vi "Load Controls.vi"(8 "Parent Label":string, 9 "Parent Class":string, 10 "Controls[]":refnum<vi>[](array[refnum]), 11 "Ref Config File In":T1) -> (3 "Ref Config File Out":T1)   [LabVIEW 2009]
uses:
  <vilib>/Utility/config.llb/Config Data RefNum.ctl
  <vilib>/Utility/config.llb/Read Key (Double).vi
  <vilib>/Utility/config.llb/Read Key (Boolean).vi
  <vilib>/Utility/config.llb/Read Key (String).vi
  <vilib>/Utility/config.llb/Read Key (Path).vi
  <vilib>/Utility/config.llb/Read Key (I32).vi
  <vilib>/Utility/config.llb/NI_LVConfig.lvlib
panel:
  # "Guillaume Plateau - Dec. 9, 2009\nyguig2@yahoo.fr - Version 3.0"
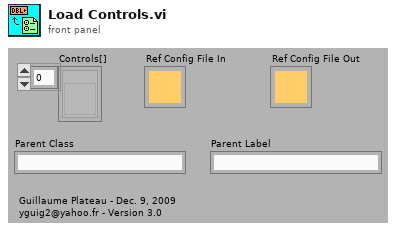
[diagram p1: front panel]
types:
  T1 = typedef "NI_LVConfig.lvlib/Config Data RefNum.ctl" = refnum<k1>
  T2 = typedef "LVCursorListTypeDef.ctl" = cluster{"Name":string, "Color":u32, "Style":u8, "Point Style":u8, "Name Visible":bool, "Allow Drag":bool, "Cursor Mode":u32, "Plot":i32, "Index":i32, "Position":cluster{"X":dbl, "Y":dbl}, "X Scale":u32, "Y Scale":u32, "Watch Plots":i32[], "Watch All Plots":bool, "Plot Area":i32, "Label Offset":cluster{"X":dbl, "Y":dbl}}[]
  T3 = cluster{"Name":string, "Color":u32, "Style":u8, "Point Style":u8, "Name Visible":bool, "Allow Drag":bool, "Cursor Mode":u32, "Plot":i32, "Index":i32, "Position":cluster{"X":dbl, "Y":dbl}, "X Scale":u32, "Y Scale":u32, "Watch Plots":i32[], "Watch All Plots":bool, "Plot Area":i32, "Label Offset":cluster{"X":dbl, "Y":dbl}}
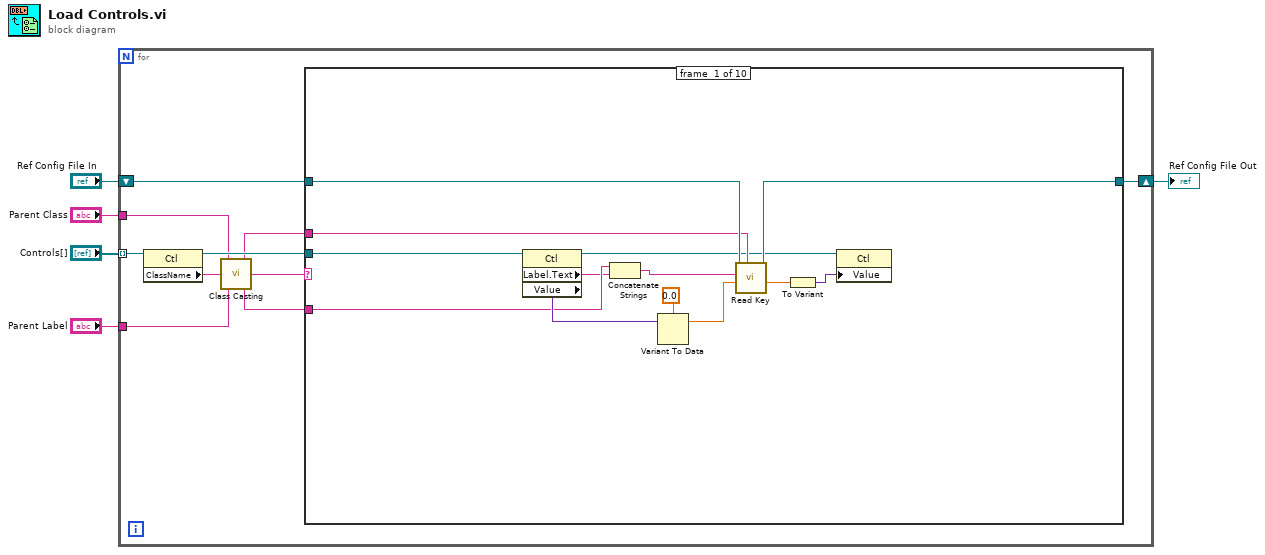
[diagram p0: block diagram]
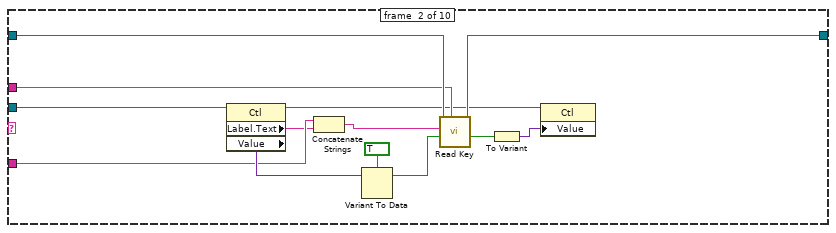
[diagram p2: hidden frame]
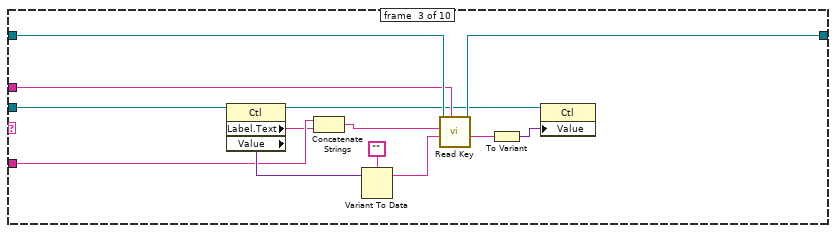
[diagram p3: hidden frame]
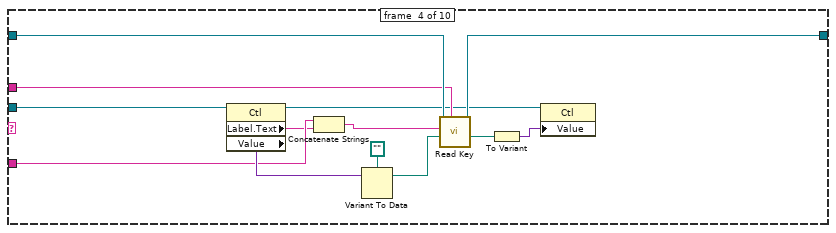
[diagram p4: hidden frame]
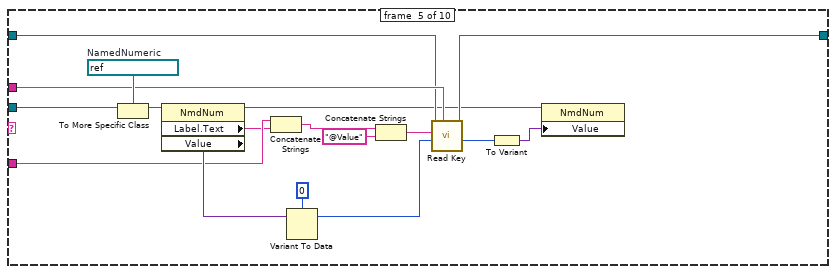
[diagram p5: hidden frame]
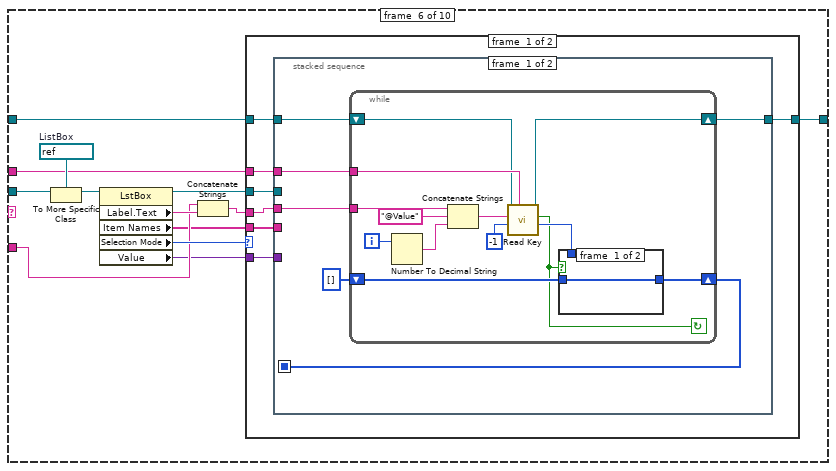
[diagram p6: hidden frame]
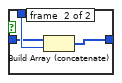
[diagram p7: hidden frame]
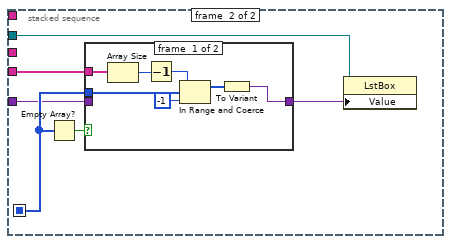
[diagram p8: hidden frame]
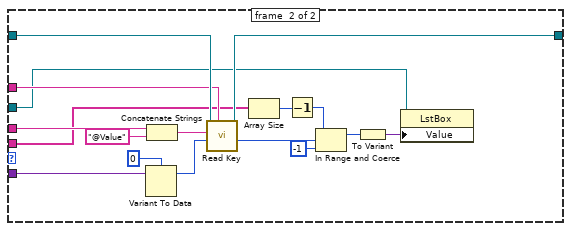
[diagram p10: hidden frame]
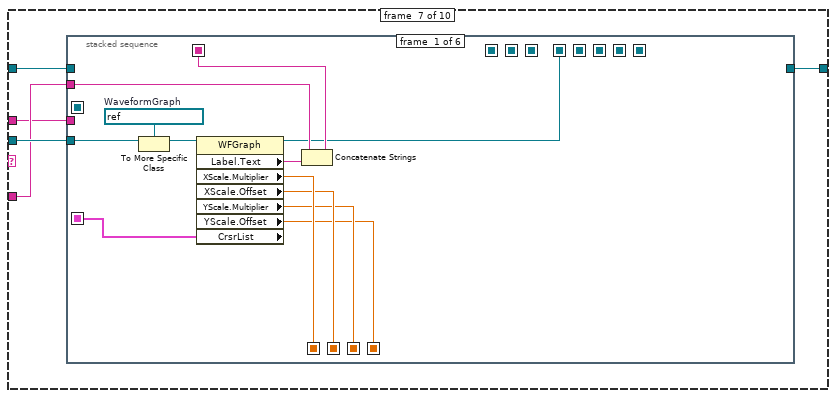
[diagram p11: hidden frame]
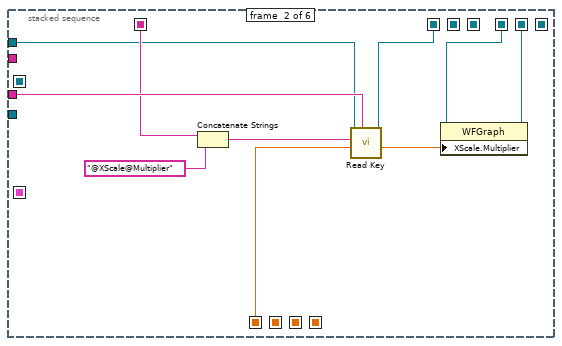
[diagram p12: hidden frame]
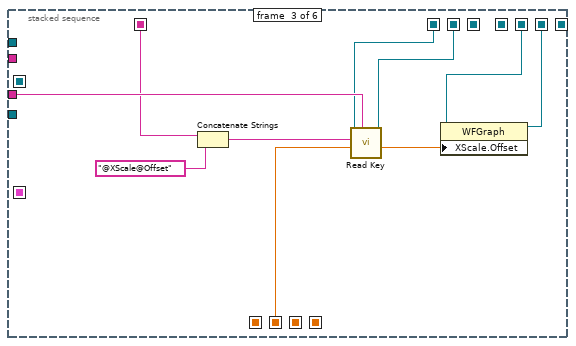
[diagram p13: hidden frame]
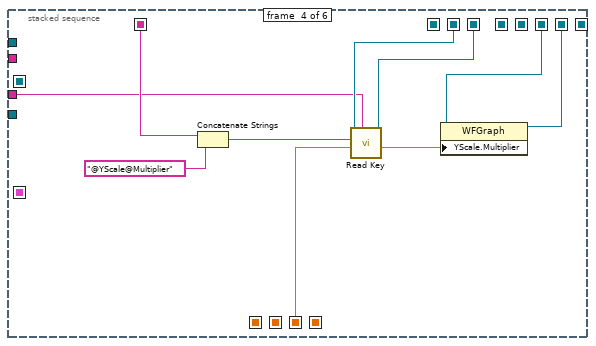
[diagram p14: hidden frame]
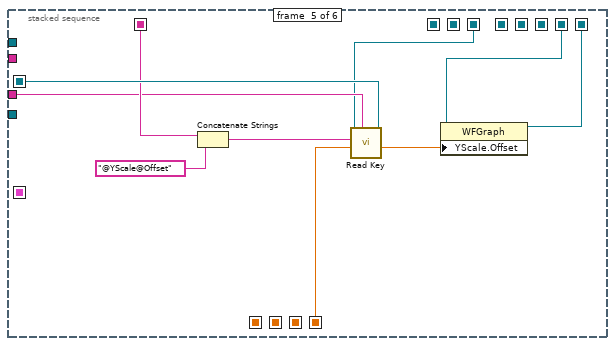
[diagram p15: hidden frame]
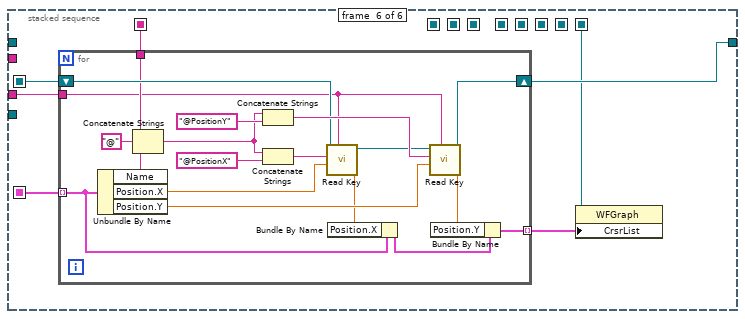
[diagram p16: hidden frame]
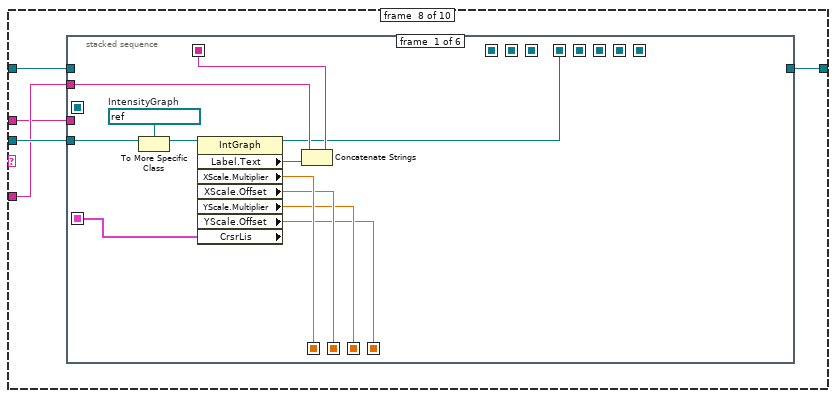
[diagram p17: hidden frame]
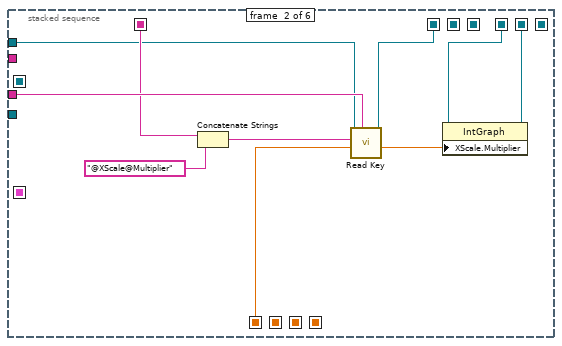
[diagram p18: hidden frame]
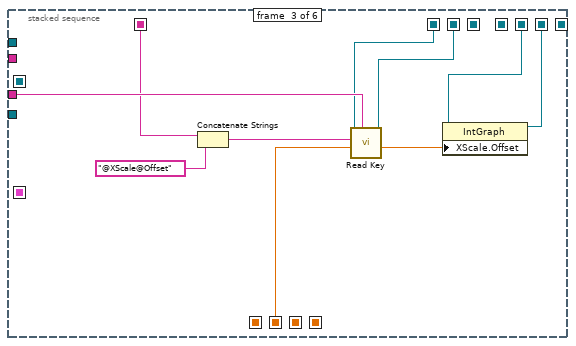
[diagram p19: hidden frame]
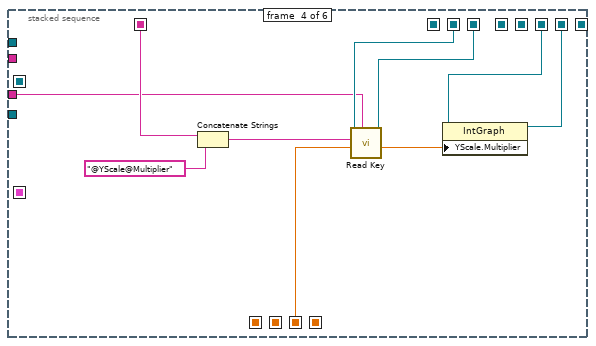
[diagram p20: hidden frame]
diagram:
  n1 = for {
    tunnel: "Controls[]" -> [w12] mode=indexing
    shift-right: [w13] -> w5
    shift-left: "Ref Config File In" -> [w14]
    tunnel: "Parent Class" -> [w7]
    tunnel: "Parent Label" -> [w11]
    n2 = property class="Ctl"(reference=w12) -> (reference out=w9:refnum<vi>, "ClassName"=w8:string)  [unwired: 1 in, 1 out]
    n3 = call "Class Casting.vi"("Parent Label"=w11, "Control Class"=w8, "Parent Class"=w7) -> ("Add-on Label"=w10:string, "Class"=w6:string)  [unwired: 1 out]
    n4 = case shown="\"WaveformGraph\"" w8 {
      tunnel: w9 -> [w15 w39 w52 w65 w82 w96 w162 w245 w328 _]
      tunnel: w14 -> [w25 w37 w50 w63 w71 w92 w161 w244 w327 w407]
      tunnel: [w24 w36 w49 w62 w83 w91 w160 w243 w326 w407] -> w13
      tunnel: w10 -> [w23 w34 w47 w60 w75 w88 w159 w242 w325 _]
      tunnel: w6 -> [w20 w32 w45 w58 w72 w87 w158 w241 w324 _]
      frame #0 {
        n5 = property class="Ctl"(reference=w15) -> (reference out=w18:refnum<vi>, "Label.Text"=w21:string, "Value"=w26:variant)  [unwired: 1 in, 1 out]
        n6 = Concatenate Strings(w23, w21) -> (w22:string)
        n7 = Variant To Data(Variant=w26, type=0.0) -> (data=w19:dbl)  [unwired: 1 in, 1 out]
        n8 = call-poly <vilib>:"Read Key.vi"("section"=w20, "default value"=w19, "key"=w22, "refnum"=w25) -> ("value"=w17:dbl, "refnum out"=w24:T1)  [unwired: 3 in, 3 out]
        n9 = To Variant(anything=w17) -> (Variant=w16:variant)
        n10 = property class="Ctl"(reference=w18, "Value"=w16) -> ()  [unwired: 1 in, 2 out]
      }
      frame #1 {
        n11 = property class="Ctl"(reference=w39) -> (reference out=w28:refnum<vi>, "Label.Text"=w33:string, "Value"=w38:variant)  [unwired: 1 in, 1 out]
        n12 = Concatenate Strings(w34, w33) -> (w35:string)
        n13 = Variant To Data(Variant=w38, type=TRUE) -> (data=w31:bool)  [unwired: 1 in, 1 out]
        n14 = call-poly <vilib>:"Read Key.vi"("section"=w32, "default value"=w31, "key"=w35, "refnum"=w37) -> ("value"=w29:bool, "refnum out"=w36:T1)  [unwired: 1 in, 5 out]
        n15 = To Variant(anything=w29) -> (Variant=w30:variant)
        n16 = property class="Ctl"(reference=w28, "Value"=w30) -> ()  [unwired: 1 in, 2 out]
      }
      frame #2 {
        n17 = property class="Ctl"(reference=w52) -> (reference out=w41:refnum<vi>, "Label.Text"=w46:string, "Value"=w51:variant)  [unwired: 1 in, 1 out]
        n18 = Concatenate Strings(w47, w46) -> (w48:string)
        n19 = Variant To Data(Variant=w51, type="") -> (data=w44:string)  [unwired: 1 in, 1 out]
        n20 = call-poly <vilib>:"Read Key.vi"("section"=w45, "default value"=w44, "key"=w48, "refnum"=w50) -> ("value"=w42:string, "refnum out"=w49:T1)  [unwired: 2 in, 4 out]
        n21 = To Variant(anything=w42) -> (Variant=w43:variant)
        n22 = property class="Ctl"(reference=w41, "Value"=w43) -> ()  [unwired: 1 in, 2 out]
      }
      frame #3 {
        n23 = property class="Ctl"(reference=w65) -> (reference out=w54:refnum<vi>, "Label.Text"=w59:string, "Value"=w64:variant)  [unwired: 1 in, 1 out]
        n24 = Concatenate Strings(w60, w59) -> (w61:string)
        n25 = Variant To Data(Variant=w64, type=path "") -> (data=w57:path)  [unwired: 1 in, 1 out]
        n26 = call-poly <vilib>:"Read Key.vi"("section"=w58, "default value"=w57, "key"=w61, "refnum"=w63) -> ("value"=w55:path, "refnum out"=w62:T1)  [unwired: 1 in, 5 out]
        n27 = To Variant(anything=w55) -> (Variant=w56:variant)
        n28 = property class="Ctl"(reference=w54, "Value"=w56) -> ()  [unwired: 1 in, 2 out]
      }
      frame #4 {
        w81 = refnum<vi> refnum  # NamedNumeric
        n29 = To More Specific Class(target class=w81, reference=w82) -> (specific class reference=w80:refnum<vi>)  [unwired: 1 in, 1 out]
        n30 = property class="NmdNum"(reference=w80) -> (reference out=w67:refnum<vi>, "Label.Text"=w74:string, "Value"=w78:variant)  [unwired: 1 in, 1 out]
        n31 = Concatenate Strings(w75, w74) -> (w73:string)
        n32 = Variant To Data(Variant=w78, type=0) -> (data=w69:i32)  [unwired: 1 in, 1 out]
        n33 = Concatenate Strings(w73, "@Value" ("string")) -> (w76:string)
        n34 = call-poly <vilib>:"Read Key.vi"("section"=w72, "default value"=w69, "key"=w76, "refnum"=w71) -> ("value"=w68:i32, "refnum out"=w83:T1)  [unwired: 1 in, 5 out]
        n35 = To Variant(anything=w68) -> (Variant=w70:variant)
        n36 = property class="NmdNum"(reference=w67, "Value"=w70) -> ()  [unwired: 1 in, 2 out]
      }
      frame #5 {
        w95 = refnum<vi> refnum  # ListBox
        n37 = To More Specific Class(target class=w95, reference=w96) -> (specific class reference=w94:refnum<vi>)  [unwired: 1 in, 1 out]
        n38 = property class="LstBox"(reference=w94) -> (reference out=w85:refnum<vi>, "Label.Text"=w90:string, "Item Names"=w86:string[], "Selection Mode"=w93:i32, "Value"=w84:variant)  [unwired: 1 in, 1 out]
        n39 = Concatenate Strings(w88, w90) -> (w89:string)
        n40 = case shown="0, 1, Default" w93 {
          tunnel: w92 -> [w103 w157]
          tunnel: w87 -> [w102 w156]
          tunnel: w89 -> [w101 w155]
          tunnel: [w100 w154] -> w91
          tunnel: w86 -> [w99 w143]
          tunnel: w85 -> [w97 w141]
          tunnel: w84 -> [w98 w150]
          frame #0 {
            n41 = stacked-sequence {
              seq-local: [w104 _] -> [_ w131]
              tunnel: w103 -> [w109 _]
              tunnel: w102 -> [w108 _]
              tunnel: w101 -> [w107 _]
              tunnel: [w106 _] -> w100
              tunnel: w99 -> [_ w130]
              tunnel: w98 -> [_ w129]
              tunnel: w97 -> [_ w127]
              frame #0 {
                n42 = while {
                  shift-right: [w118] -> w106
                  shift-left: w109 -> [w115]
                  tunnel: w108 -> [w116]
                  tunnel: w107 -> [w117]
                  shift-right: [w111] -> w104
                  shift-left: i32[] [] -> [w112]
                  i -> [w120]
                  stop <- w110 continue-if-true
                  n43 = Number To Decimal String(number=w120) -> (decimal integer string=w119:string)  [unwired: 1 out]
                  n44 = Concatenate Strings(w117, "@Value" ("string"), w119) -> (w121:string)
                  n45 = call-poly <vilib>:"Read Key.vi"("section"=w116, "default value"=-1, "key"=w121, "refnum"=w115) -> ("value"=w113:i32, "found?"=w110:bool, "refnum out"=w118:T1)  [unwired: 1 in, 4 out]
                  n46 = case shown="True" w110 {
                    tunnel: w113 -> [_ w126]
                    tunnel: w112 -> [w123 w125]
                    tunnel: [w123 w124] -> w111
                    frame #0 {
                    }
                    frame #1 {
                      n47 = Build Array (concatenate)(w125, w126) -> (w124:i32[])
                    }
                  }
                }
              }
              frame #1 {
                n48 = Empty Array?(array=w131) -> (empty?=w132:bool)
                n49 = case shown="False" w132 {
                  tunnel: w131 -> [w135 _]
                  tunnel: w130 -> [w134 _]
                  tunnel: [w133 w140] -> w128
                  tunnel: w129 -> [_ w140]
                  frame #0 {
                    n50 = Array Size(array=w134) -> (size(s)=w138:i32)
                    n51 = Decrement(x=w138) -> (x-1=w137:i32)
                    n52 = In Range and Coerce(upper limit=w137, x=w135, lower limit=-1) -> (coerced(x)=w136:i32[])  [unwired: 1 out]
                    n53 = To Variant(anything=w136) -> (Variant=w133:variant)
                  }
                  frame #1 {
                  }
                }
                n54 = property class="LstBox"(reference=w127, "Value"=w128) -> ()  [unwired: 1 in, 2 out]
              }
            }
          }
          frame #1 {
            n55 = Variant To Data(Variant=w150, type=0) -> (data=w149:i32)  [unwired: 1 in, 1 out]
            n56 = Concatenate Strings(w155, "@Value" ("string")) -> (w152:string)
            n57 = call-poly <vilib>:"Read Key.vi"("section"=w156, "default value"=w149, "key"=w152, "refnum"=w157) -> ("value"=w144:i32, "refnum out"=w154:T1)  [unwired: 1 in, 5 out]
            n58 = Array Size(array=w143) -> (size(s)=w147:i32)
            n59 = Decrement(x=w147) -> (x-1=w146:i32)
            n60 = In Range and Coerce(upper limit=w146, x=w144, lower limit=-1) -> (coerced(x)=w145:i32)  [unwired: 1 out]
            n61 = To Variant(anything=w145) -> (Variant=w142:variant)
            n62 = property class="LstBox"(reference=w141, "Value"=w142) -> ()  [unwired: 1 in, 2 out]
          }
        }
      }
      frame #6 {
        n63 = stacked-sequence {
          seq-local: [w171 _ _ _ _ _] -> [_ _ _ _ _ w221]
          seq-local: [_ _ _ _ w212 _] -> [_ _ _ _ _ w220]
          seq-local: [w170 _ _ _ _ _] -> [_ w180 _ _ _ _]
          seq-local: [w169 _ _ _ _ _] -> [_ _ w189 _ _ _]
          seq-local: [w168 _ _ _ _ _] -> [_ _ _ w198 _ _]
          seq-local: [w167 _ _ _ _ _] -> [_ _ _ _ w209 _]
          seq-local: [_ w176 _ _ _ _] -> [_ _ w188 _ _ _]
          seq-local: [_ _ w192 _ _ _] -> [_ _ _ w202 _ _]
          seq-local: [_ _ _ w201 _ _] -> [_ _ _ _ w206 _]
          seq-local: [w164 _ _ _ _ _] -> [_ w181 w190 w200 w211 w218]
          seq-local: [w163 _ _ _ _ _] -> [_ w175 _ _ _ _]
          seq-local: [_ w177 _ _ _ _] -> [_ _ w187 _ _ _]
          seq-local: [_ _ w185 _ _ _] -> [_ _ _ w197 _ _]
          seq-local: [_ _ _ w195 _ _] -> [_ _ _ _ w205 _]
          seq-local: [_ _ _ _ w207 _] -> [_ _ _ _ _ w215]
          tunnel: w162 -> [w172 _ _ _ _ _]
          tunnel: w161 -> [_ w178 _ _ _ _]
          tunnel: [_ _ _ _ _ w219] -> w160
          tunnel: w158 -> [_ w182 w191 w199 w210 w217]
          tunnel: w159 -> [w165 _ _ _ _ _]
          frame #0 {
            w174 = refnum<vi> refnum  # WaveformGraph
            n64 = To More Specific Class(target class=w174, reference=w172) -> (specific class reference=w173:refnum<vi>)  [unwired: 1 in, 1 out]
            n65 = property class="WFGraph"(reference=w173) -> (reference out=w163:refnum<vi>, "Label.Text"=w166:string, "XScale.Multiplier"=w170:dbl, "XScale.Offset"=w169:dbl, "YScale.Multiplier"=w168:dbl, "YScale.Offset"=w167:dbl, "CrsrList"=w171:T2)  [unwired: 1 in, 1 out]
            n66 = Concatenate Strings(w165, w166) -> (w164:string)
          }
          frame #1 {
            n67 = Concatenate Strings(w181, "@XScale@Multiplier" ("string")) -> (w183:string)
            n68 = call-poly <vilib>:"Read Key.vi"("section"=w182, "default value"=w180, "key"=w183, "refnum"=w178) -> ("value"=w179:dbl, "refnum out"=w176:T1)  [unwired: 1 in, 5 out]
            n69 = property class="WFGraph"(reference=w175, "XScale.Multiplier"=w179) -> (reference out=w177:refnum<vi>)  [unwired: 1 in, 1 out]
          }
          frame #2 {
            n70 = Concatenate Strings(w190, "@XScale@Offset" ("string")) -> (w193:string)
            n71 = call-poly <vilib>:"Read Key.vi"("section"=w191, "default value"=w189, "key"=w193, "refnum"=w188) -> ("value"=w186:dbl, "refnum out"=w192:T1)  [unwired: 1 in, 5 out]
            n72 = property class="WFGraph"(reference=w187, "XScale.Offset"=w186) -> (reference out=w185:refnum<vi>)  [unwired: 1 in, 1 out]
          }
          frame #3 {
            n73 = Concatenate Strings(w200, "@YScale@Multiplier" ("string")) -> (w203:string)
            n74 = call-poly <vilib>:"Read Key.vi"("section"=w199, "default value"=w198, "key"=w203, "refnum"=w202) -> ("value"=w196:dbl, "refnum out"=w201:T1)  [unwired: 1 in, 5 out]
            n75 = property class="WFGraph"(reference=w197, "YScale.Multiplier"=w196) -> (reference out=w195:refnum<vi>)  [unwired: 1 in, 1 out]
          }
          frame #4 {
            n76 = Concatenate Strings(w211, "@YScale@Offset" ("string")) -> (w213:string)
            n77 = call-poly <vilib>:"Read Key.vi"("section"=w210, "default value"=w209, "key"=w213, "refnum"=w206) -> ("value"=w208:dbl, "refnum out"=w212:T1)  [unwired: 1 in, 5 out]
            n78 = property class="WFGraph"(reference=w205, "YScale.Offset"=w208) -> (reference out=w207:refnum<vi>)  [unwired: 1 in, 1 out]
          }
          frame #5 {
            n79 = for {
              shift-right: [w231] -> w219
              shift-left: w220 -> [w232]
              tunnel: w221 -> [w224] mode=indexing
              tunnel: w218 -> [w230]
              tunnel: w217 -> [w229]
              tunnel: [w222] -> w216 mode=indexing
              n80 = Unbundle By Name(w224) -> ("Name"=w239:string, "Position.X"=w228:dbl, "Position.Y"=w227:dbl)
              n81 = Concatenate Strings(w230, "@" ("string"), w239) -> (w233:string)
              n82 = Concatenate Strings(w233, "@PositionY" ("string")) -> (w235:string)
              n83 = Concatenate Strings(w233, "@PositionX" ("string")) -> (w236:string)
              n84 = call-poly <vilib>:"Read Key.vi"("section"=w229, "default value"=w228, "key"=w236, "refnum"=w232) -> ("value"=w226:dbl, "refnum out"=w234:T1)  [unwired: 1 in, 5 out]
              n85 = Bundle By Name(cluster=w224, "Position.X"=w226) -> (w223:T3)
              n86 = call-poly <vilib>:"Read Key.vi"("section"=w229, "default value"=w227, "key"=w235, "refnum"=w234) -> ("value"=w225:dbl, "refnum out"=w231:T1)  [unwired: 1 in, 5 out]
              n87 = Bundle By Name(cluster=w223, "Position.Y"=w225) -> (w222:T3)
            }
            n88 = property class="WFGraph"(reference=w215, "CrsrList"=w216) -> ()  [unwired: 1 in, 2 out]
          }
        }
      }
      frame #7 {
        n89 = stacked-sequence {
          seq-local: [w254 _ _ _ _ _] -> [_ _ _ _ _ w304]
          seq-local: [_ _ _ _ w295 _] -> [_ _ _ _ _ w303]
          seq-local: [w253 _ _ _ _ _] -> [_ w263 _ _ _ _]
          seq-local: [w252 _ _ _ _ _] -> [_ _ w272 _ _ _]
          seq-local: [w251 _ _ _ _ _] -> [_ _ _ w281 _ _]
          seq-local: [w250 _ _ _ _ _] -> [_ _ _ _ w292 _]
          seq-local: [_ w259 _ _ _ _] -> [_ _ w271 _ _ _]
          seq-local: [_ _ w275 _ _ _] -> [_ _ _ w285 _ _]
          seq-local: [_ _ _ w284 _ _] -> [_ _ _ _ w289 _]
          seq-local: [w247 _ _ _ _ _] -> [_ w264 w273 w283 w294 w301]
          seq-local: [w246 _ _ _ _ _] -> [_ w258 _ _ _ _]
          seq-local: [_ w260 _ _ _ _] -> [_ _ w270 _ _ _]
          seq-local: [_ _ w268 _ _ _] -> [_ _ _ w280 _ _]
          seq-local: [_ _ _ w278 _ _] -> [_ _ _ _ w288 _]
          seq-local: [_ _ _ _ w290 _] -> [_ _ _ _ _ w298]
          tunnel: w245 -> [w255 _ _ _ _ _]
          tunnel: w244 -> [_ w261 _ _ _ _]
          tunnel: [_ _ _ _ _ w302] -> w243
          tunnel: w241 -> [_ w265 w274 w282 w293 w300]
          tunnel: w242 -> [w248 _ _ _ _ _]
          frame #0 {
            w257 = refnum<vi> refnum  # IntensityGraph
            n90 = To More Specific Class(target class=w257, reference=w255) -> (specific class reference=w256:refnum<vi>)  [unwired: 1 in, 1 out]
            n91 = property class="IntGraph"(reference=w256) -> (reference out=w246:refnum<vi>, "Label.Text"=w249:string, "XScale.Multiplier"=w253:dbl, "XScale.Offset"=w252:dbl, "YScale.Multiplier"=w251:dbl, "YScale.Offset"=w250:dbl, "CrsrLis"=w254:T2)  [unwired: 1 in, 1 out]
            n92 = Concatenate Strings(w248, w249) -> (w247:string)
          }
          frame #1 {
            n93 = Concatenate Strings(w264, "@XScale@Multiplier" ("string")) -> (w266:string)
            n94 = call-poly <vilib>:"Read Key.vi"("section"=w265, "default value"=w263, "key"=w266, "refnum"=w261) -> ("value"=w262:dbl, "refnum out"=w259:T1)  [unwired: 1 in, 5 out]
            n95 = property class="IntGraph"(reference=w258, "XScale.Multiplier"=w262) -> (reference out=w260:refnum<vi>)  [unwired: 1 in, 1 out]
          }
          frame #2 {
            n96 = Concatenate Strings(w273, "@XScale@Offset" ("string")) -> (w276:string)
            n97 = call-poly <vilib>:"Read Key.vi"("section"=w274, "default value"=w272, "key"=w276, "refnum"=w271) -> ("value"=w269:dbl, "refnum out"=w275:T1)  [unwired: 1 in, 5 out]
            n98 = property class="IntGraph"(reference=w270, "XScale.Offset"=w269) -> (reference out=w268:refnum<vi>)  [unwired: 1 in, 1 out]
          }
          frame #3 {
            n99 = Concatenate Strings(w283, "@YScale@Multiplier" ("string")) -> (w286:string)
            n100 = call-poly <vilib>:"Read Key.vi"("section"=w282, "default value"=w281, "key"=w286, "refnum"=w285) -> ("value"=w279:dbl, "refnum out"=w284:T1)  [unwired: 1 in, 5 out]
            n101 = property class="IntGraph"(reference=w280, "YScale.Multiplier"=w279) -> (reference out=w278:refnum<vi>)  [unwired: 1 in, 1 out]
          }
          frame #4 {
            n102 = Concatenate Strings(w294, "@YScale@Offset" ("string")) -> (w296:string)
            n103 = call-poly <vilib>:"Read Key.vi"("section"=w293, "default value"=w292, "key"=w296, "refnum"=w289) -> ("value"=w291:dbl, "refnum out"=w295:T1)  [unwired: 1 in, 5 out]
            n104 = property class="IntGraph"(reference=w288, "YScale.Offset"=w291) -> (reference out=w290:refnum<vi>)  [unwired: 1 in, 1 out]
          }
          frame #5 {
            n105 = for {
              shift-right: [w314] -> w302
              shift-left: w303 -> [w315]
              tunnel: w304 -> [w307] mode=indexing
              tunnel: w301 -> [w313]
              tunnel: w300 -> [w312]
              tunnel: [w305] -> w299 mode=indexing
              n106 = Unbundle By Name(w307) -> ("Name"=w322:string, "Position.X"=w311:dbl, "Position.Y"=w310:dbl)
              n107 = Concatenate Strings(w313, "@" ("string"), w322) -> (w316:string)
              n108 = Concatenate Strings(w316, "@PositionY" ("string")) -> (w318:string)
              n109 = Concatenate Strings(w316, "@PositionX" ("string")) -> (w319:string)
              n110 = call-poly <vilib>:"Read Key.vi"("section"=w312, "default value"=w311, "key"=w319, "refnum"=w315) -> ("value"=w309:dbl, "refnum out"=w317:T1)  [unwired: 1 in, 5 out]
              n111 = Bundle By Name(cluster=w307, "Position.X"=w309) -> (w306:T3)
              n112 = call-poly <vilib>:"Read Key.vi"("section"=w312, "default value"=w310, "key"=w318, "refnum"=w317) -> ("value"=w308:dbl, "refnum out"=w314:T1)  [unwired: 1 in, 5 out]
              n113 = Bundle By Name(cluster=w306, "Position.Y"=w308) -> (w305:T3)
            }
            n114 = property class="IntGraph"(reference=w298, "CrsrLis"=w299) -> ()  [unwired: 1 in, 2 out]
          }
        }
      }
      frame #8 {
        n115 = stacked-sequence {
          seq-local: [w337 _ _ _ _ _] -> [_ _ _ _ _ w387]
          seq-local: [_ _ _ _ w378 _] -> [_ _ _ _ _ w386]
          seq-local: [w336 _ _ _ _ _] -> [_ w346 _ _ _ _]
          seq-local: [w335 _ _ _ _ _] -> [_ _ w355 _ _ _]
          seq-local: [w334 _ _ _ _ _] -> [_ _ _ w364 _ _]
          seq-local: [w333 _ _ _ _ _] -> [_ _ _ _ w375 _]
          seq-local: [_ w342 _ _ _ _] -> [_ _ w354 _ _ _]
          seq-local: [_ _ w358 _ _ _] -> [_ _ _ w368 _ _]
          seq-local: [_ _ _ w367 _ _] -> [_ _ _ _ w372 _]
          seq-local: [w330 _ _ _ _ _] -> [_ w347 w356 w366 w377 w384]
          seq-local: [w329 _ _ _ _ _] -> [_ w341 _ _ _ _]
          seq-local: [_ w343 _ _ _ _] -> [_ _ w353 _ _ _]
          seq-local: [_ _ w351 _ _ _] -> [_ _ _ w363 _ _]
          seq-local: [_ _ _ w361 _ _] -> [_ _ _ _ w371 _]
          seq-local: [_ _ _ _ w373 _] -> [_ _ _ _ _ w381]
          tunnel: w328 -> [w338 _ _ _ _ _]
          tunnel: w327 -> [_ w344 _ _ _ _]
          tunnel: [_ _ _ _ _ w385] -> w326
          tunnel: w324 -> [_ w348 w357 w365 w376 w383]
          tunnel: w325 -> [w331 _ _ _ _ _]
          frame #0 {
            w340 = refnum<vi> refnum  # XYGraph
            n116 = To More Specific Class(target class=w340, reference=w338) -> (specific class reference=w339:refnum<vi>)  [unwired: 1 in, 1 out]
            n117 = property class="XYGraph"(reference=w339) -> (reference out=w329:refnum<vi>, "Label.Text"=w332:string, "XScale.Multiplier"=w336:dbl, "XScale.Offset"=w335:dbl, "YScale.Multiplier"=w334:dbl, "YScale.Offset"=w333:dbl, "CrsrList"=w337:T2)  [unwired: 1 in, 1 out]
            n118 = Concatenate Strings(w331, w332) -> (w330:string)
          }
          frame #1 {
            n119 = Concatenate Strings(w347, "@XScale@Multiplier" ("string")) -> (w349:string)
            n120 = call-poly <vilib>:"Read Key.vi"("section"=w348, "default value"=w346, "key"=w349, "refnum"=w344) -> ("value"=w345:dbl, "refnum out"=w342:T1)  [unwired: 1 in, 5 out]
            n121 = property class="XYGraph"(reference=w341, "XScale.Multiplier"=w345) -> (reference out=w343:refnum<vi>)  [unwired: 1 in, 1 out]
          }
          frame #2 {
            n122 = Concatenate Strings(w356, "@XScale@Offset" ("string")) -> (w359:string)
            n123 = call-poly <vilib>:"Read Key.vi"("section"=w357, "default value"=w355, "key"=w359, "refnum"=w354) -> ("value"=w352:dbl, "refnum out"=w358:T1)  [unwired: 1 in, 5 out]
            n124 = property class="XYGraph"(reference=w353, "XScale.Offset"=w352) -> (reference out=w351:refnum<vi>)  [unwired: 1 in, 1 out]
          }
          frame #3 {
            n125 = Concatenate Strings(w366, "@YScale@Multiplier" ("string")) -> (w369:string)
            n126 = call-poly <vilib>:"Read Key.vi"("section"=w365, "default value"=w364, "key"=w369, "refnum"=w368) -> ("value"=w362:dbl, "refnum out"=w367:T1)  [unwired: 1 in, 5 out]
            n127 = property class="XYGraph"(reference=w363, "YScale.Multiplier"=w362) -> (reference out=w361:refnum<vi>)  [unwired: 1 in, 1 out]
          }
          frame #4 {
            n128 = Concatenate Strings(w377, "@YScale@Offset" ("string")) -> (w379:string)
            n129 = call-poly <vilib>:"Read Key.vi"("section"=w376, "default value"=w375, "key"=w379, "refnum"=w372) -> ("value"=w374:dbl, "refnum out"=w378:T1)  [unwired: 1 in, 5 out]
            n130 = property class="XYGraph"(reference=w371, "YScale.Offset"=w374) -> (reference out=w373:refnum<vi>)  [unwired: 1 in, 1 out]
          }
          frame #5 {
            n131 = for {
              shift-right: [w397] -> w385
              shift-left: w386 -> [w398]
              tunnel: w387 -> [w390] mode=indexing
              tunnel: w384 -> [w396]
              tunnel: w383 -> [w395]
              tunnel: [w388] -> w382 mode=indexing
              n132 = Unbundle By Name(w390) -> ("Name"=w405:string, "Position.X"=w394:dbl, "Position.Y"=w393:dbl)
              n133 = Concatenate Strings(w396, "@" ("string"), w405) -> (w399:string)
              n134 = Concatenate Strings(w399, "@PositionY" ("string")) -> (w401:string)
              n135 = Concatenate Strings(w399, "@PositionX" ("string")) -> (w402:string)
              n136 = call-poly <vilib>:"Read Key.vi"("section"=w395, "default value"=w394, "key"=w402, "refnum"=w398) -> ("value"=w392:dbl, "refnum out"=w400:T1)  [unwired: 1 in, 5 out]
              n137 = Bundle By Name(cluster=w390, "Position.X"=w392) -> (w389:T3)
              n138 = call-poly <vilib>:"Read Key.vi"("section"=w395, "default value"=w393, "key"=w401, "refnum"=w400) -> ("value"=w391:dbl, "refnum out"=w397:T1)  [unwired: 1 in, 5 out]
              n139 = Bundle By Name(cluster=w389, "Position.Y"=w391) -> (w388:T3)
            }
            n140 = property class="XYGraph"(reference=w381, "CrsrList"=w382) -> ()  [unwired: 1 in, 2 out]
          }
        }
      }
      frame #9 {
      }
    }
  }
  "Ref Config File Out" <- w5
